vi "Write Serial Configuration.vi"(8 "error in (no error)":errorcluster, 10 "Serial Configuration":T1 {"parity" items=["None", "Odd", "Even", "Mark", "Space"]; "stopBits" items=["None", "One", "Two", "OnePointFive"]}, 11 "InovanceSerialModbusRtu in":refnum<class "InovanceSerialModbusRtu.lvclass">) -> (0 "error out":errorcluster, 3 "InovanceSerialModbusRtu out":refnum<class "InovanceSerialModbusRtu.lvclass">)   [LabVIEW 2020, in "HslCommunication.lvlib" / "InovanceSerialModbusRtu.lvclass"]
uses:
  InovanceSerialModbusRtu.lvclass
  InovanceSerialModbusRtu.lvclass/InovanceSerialModbusRtu.ctl
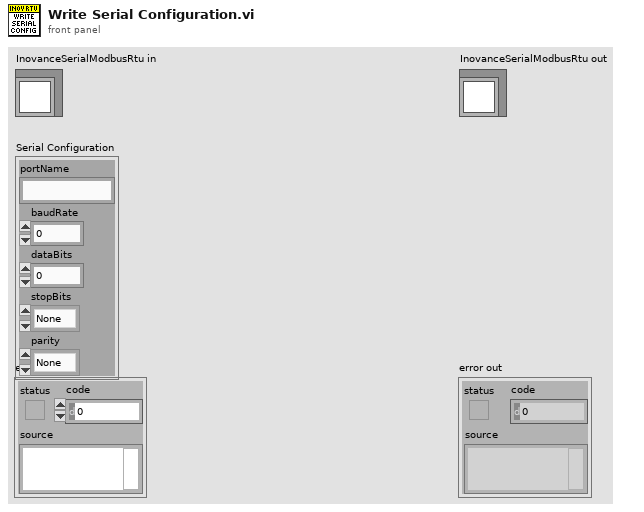
[diagram p1: front panel]
types:
  T1 = cluster{"portName":string, "baudRate":i32, "dataBits":i32, "stopBits":i32, "parity":i32}
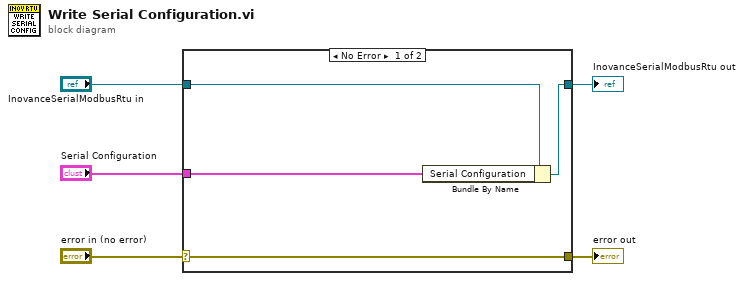
[diagram p0: block diagram]
diagram:
  n1 = case shown="No Error" "error in (no error)" {
    selector: "error in (no error)" -> [w9 w10]
    tunnel: [w9 w10] -> w4
    tunnel: [w7 w11] -> w2
    tunnel: "InovanceSerialModbusRtu in" -> [w8 w11]
    tunnel: "Serial Configuration" -> [w6 _]
    frame No Error {
      n2 = Bundle By Name(cluster=w8, "Serial Configuration"=w6) -> (w7:refnum<class "InovanceSerialModbusRtu.lvclass">)
    }
    frame Error {
    }
  }
  "error out" <- w4
  "InovanceSerialModbusRtu out" <- w2
